vi "CircularBuffer.SetSize.vi"(8 "error in (no error)":errorcluster, 10 "BufferSize":i32=1, 11 "CircularBuffer":refnum<class "CircularBuffer.lvclass">) -> (0 "error out":errorcluster, 3 "CircularBuffer out":refnum<class "CircularBuffer.lvclass">)   [LabVIEW 2013, in "CircularBuffer.lvclass"]
doc: "---------------------------------------------------------------\nJKI State Machine Objects™\nhttp://jki.net/state-machine-objects/\nCopyright (C) 2005-2015, JKI <info@jki.net>\nALL RIGHTS RESERVEDJKI State Machine Objects (SMO) 1.0.0.5\nJKI - JKI\nCopyright (c) 2016, JKI"
uses:
  CircularBuffer.lvclass
  types/type/type.lvclass
panel:
  # "For instructions on how to use the JKI State Machine Objects, examples and video tutorials, visit:\nhttp://jki.net/state-machine-objects/\n\nJKI State Machine Objects™\nhttp://jki.net/state-machine-objects/\nCopyright (C) 2005-2015, JKI <info@jki.net>\nALL RIGHTS RESERVED"
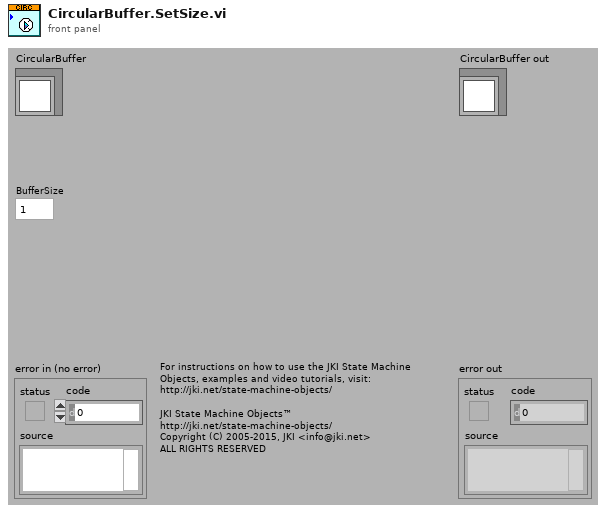
[diagram p1: front panel]
types:
  T1 = typedef "CircularBuffer.lvclass/PrivateData--Ref.ctl" = refnum<data-value>
  T2 = typedef "CircularBuffer.lvclass/PrivateData--Cluster.ctl" = cluster{"Public Events":T3, "Protected Events":T4, "Private Events":T5, "BufferSize":i32, "CurrentElement":i32, "Elements":refnum<data-value>[], "type":refnum<class "type.lvclass">}
  T3 = typedef "CircularBuffer.lvclass/PublicEvents--Cluster.ctl" = cluster{"Buffer Resize Event":refnum<user-event>}
  T4 = typedef "CircularBuffer.lvclass/ProtectedEvents--Cluster.ctl" = cluster{"placeholder":refnum<user-event>}
  T5 = typedef "CircularBuffer.lvclass/PrivateEvents--Cluster.ctl" = cluster{"New Value":refnum<user-event>, "GetElement":refnum<user-event>}
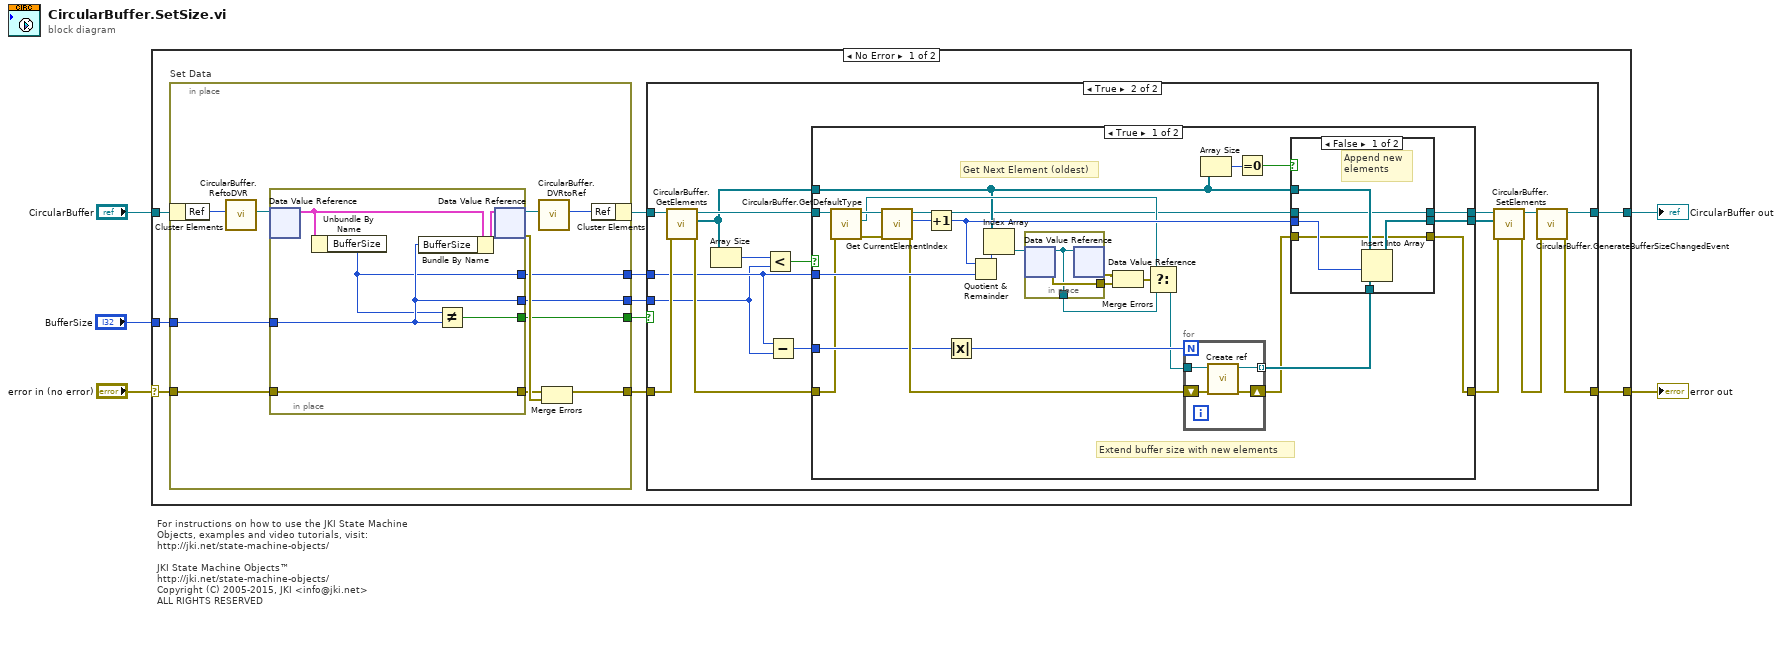
[diagram p0: block diagram]
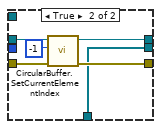
[diagram p3: hidden frame]
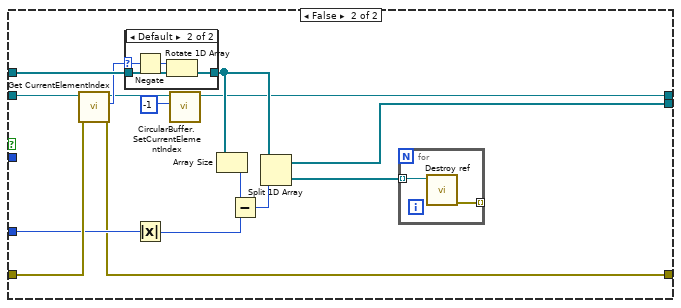
[diagram p4: hidden frame]
diagram:
  # "For instructions on how to use the JKI State Machine Objects, examples and video tutorials, visit:\nhttp://jki.net/state-machine-objects/\n\nJKI State Machine Objects™\nhttp://jki.net/state-machine-objects/\nCopyright (C) 2005-2015, JKI <info@jki.net>\nALL RIGHTS RESERVED"
  n1 = case shown="No Error" "error in (no error)" {
    selector: "error in (no error)" -> [w13 w120]
    tunnel: "CircularBuffer" -> [w14 w121]
    tunnel: [w11 w120] -> w4
    tunnel: [w9 w121] -> w3
    tunnel: "BufferSize" -> [w15 _]
    frame No Error {
      n2 = in-place "Set Data" {
        in-place-border: w13 -> [w113]
        in-place-border: [w110] -> w8
        in-place-border: w15 -> [w109]
        in-place-border: [w108] -> w12
        in-place-border: [w103] -> w7
        in-place-border: [w102] -> w6
        n3 = in-place-cluster #1(w14) -> ("Ref"=w107:u32)
        n4 = call "CircularBuffer.ReftoDVR.vi"("Ref"=w107) -> ("Ref"=w106:T1)  [unwired: 10 in]
        n5 = in-place {
          in-place-border: w113 -> [w119]
          in-place-border: [w119] -> w111
          in-place-border: w109 -> [w116]
          in-place-border: [w116] -> w108
          in-place-border: [w115] -> w103
          in-place-border: [w114] -> w102
          n6 = in-place-dvr #2(w106) -> (w117:T2)  [unwired: 1 out]
          n7 = Unbundle By Name(w117) -> ("BufferSize"=w114:i32)
          n8 = Bundle By Name(cluster=w117, "BufferSize"=w116) -> (w118:T2)
          n9 = Not Equal?(x=w114, y=w116) -> (x != y?=w115:bool)
          n10 = in-place-dvr #2(w118) -> (w105:T1, w112:errorcluster)
        }
        n11 = call "CircularBuffer.DVRtoRef.vi"("Ref"=w105) -> ("Ref"=w104:u32)  [unwired: 10 in]
        n12 = Merge Errors(w111, w112) -> (w110:errorcluster)
        n13 = in-place-cluster #1("Ref"=w104) -> (w10:refnum<class "CircularBuffer.lvclass">)
      }
      n14 = case shown="True" w7 {
        tunnel: w12 -> [_ w23]
        tunnel: [w16 w33] -> w11
        tunnel: w10 -> [w17 w32]
        tunnel: [w17 w34] -> w9
        tunnel: w8 -> [w16 w30]
        tunnel: w6 -> [_ w24]
        frame False {
        }
        frame True {
          n15 = call "CircularBuffer.GetElements.vi"("error in (no error)"=w30, "CircularBuffer in"=w32) -> ("error out"=w27:errorcluster, "Elements"=w25:refnum<data-value>[], "CircularBuffer out"=w31:refnum<class "CircularBuffer.lvclass">)  [unwired: 7 in]
          n16 = Array Size(array=w25) -> (size(s)=w29:i32)
          n17 = Less?(x=w29, y=w23) -> (x < y?=w28:bool)
          n18 = Subtract(x=w24, y=w23) -> (x-y=w22:i32)
          n19 = case shown="True" w28 {
            tunnel: [w39 w81] -> w26
            tunnel: w31 -> [w52 w94]
            tunnel: [w35 w83] -> w20
            tunnel: w27 -> [w50 w93]
            tunnel: w25 -> [w42 w91]
            tunnel: w24 -> [w61 _]
            tunnel: w22 -> [w57 w92]
            tunnel: [w55 w85] -> w21
            frame True {
              # "Get Next Element (oldest)"
              # "Extend buffer size with new elements"
              n20 = call "CircularBuffer.GetDefaultType.vi"("error in (no error)"=w50, "CircularBuffer"=w52) -> ("error out"=w49:errorcluster, "type"=w44:refnum<class "type.lvclass">, "CircularBuffer out"=w51:refnum<class "CircularBuffer.lvclass">)  [unwired: 7 in]
              n21 = call "Get CurrentElementIndex.vi"("error in (no error)"=w49, "CircularBuffer"=w51) -> ("error out"=w58:errorcluster, "Current Element index"=w53:i32, "CircularBuffer out"=w38:refnum<class "CircularBuffer.lvclass">)  [unwired: 7 in]
              n22 = Increment(x=w53) -> (x+1=w56:i32)
              n23 = Absolute Value(x=w57) -> (abs(x)=w54:i32)
              n24 = Quotient & Remainder(x=w56, y=w61) -> (x-y*floor(x/y)=w60:i32)  [unwired: 1 out]
              n25 = Index Array(array=w42, index=w60) -> (element=w59:refnum<data-value>)
              n26 = in-place {
                in-place-border: [w79] -> w47
                in-place-border: [w78] -> w45
                n27 = in-place-dvr #3(w59) -> (w78:refnum<class "type.lvclass">, w79:errorcluster)
                n28 = in-place-dvr #3(w78) -> (w48:errorcluster)  [unwired: 1 out]
              }
              n29 = Merge Errors(w48, w47) -> (w46:errorcluster)
              n30 = Select(t=w44, s=w46, f=w45) -> (s? t:f=w43:refnum<class "type.lvclass">)
              n31 = for {
                N: w54 -> [_]
                tunnel: [w75] -> w37 mode=indexing
                shift-right: [w76] -> w36
                shift-left: w58 -> [w77]
                tunnel: w43 -> [w74]
                n32 = call "Create ref.vi"("error in (no error)"=w77, "type in"=w74) -> ("error out"=w76:errorcluster, "data value reference"=w75:refnum<data-value>)  [unwired: 8 in]
              }
              n33 = Array Size(array=w42) -> (size(s)=w41:i32)
              n34 = Equal To 0?(x=w41) -> (x = 0?=w40:bool)
              n35 = case shown="False" w40 {
                tunnel: w56 -> [w67 _]
                tunnel: w37 -> [w66 w68]
                tunnel: [w65 w68] -> w55
                tunnel: w42 -> [w64 _]
                tunnel: [w63 w71] -> w39
                tunnel: w38 -> [w63 w72]
                tunnel: w36 -> [w62 w70]
                tunnel: [w62 w69] -> w35
                frame False {
                  # "Append new\nelements"
                  n36 = Insert Into Array(array=w64, index=w67, new element=w66) -> (w65:refnum<data-value>[])
                }
                frame True {
                  n37 = call "CircularBuffer.SetCurrentElementIndex.vi"("error in (no error)"=w70, "Index"=-1, "CircularBuffer"=w72) -> ("error out"=w69:errorcluster, "CircularBuffer out"=w71:refnum<class "CircularBuffer.lvclass">)  [unwired: 7 in]
                }
              }
            }
            frame False {
              n38 = call "Get CurrentElementIndex.vi"("error in (no error)"=w93, "CircularBuffer"=w94) -> ("error out"=w83:errorcluster, "Current Element index"=w90:i32, "CircularBuffer out"=w82:refnum<class "CircularBuffer.lvclass">)  [unwired: 7 in]
              n39 = case shown="Default" w90 {
                selector: w90 -> [_ w99]
                tunnel: w91 -> [w97 w101]
                tunnel: [w97 w98] -> w89
                frame -1 {
                }
                frame Default {
                  n40 = Negate(x=w99) -> (-x=w100:i32)
                  n41 = Rotate 1D Array(1:w101, 2:w100) -> (0:w98:refnum<data-value>[])
                }
              }
              n42 = Absolute Value(x=w92) -> (abs(x)=w87:i32)
              n43 = call "CircularBuffer.SetCurrentElementIndex.vi"("Index"=-1, "CircularBuffer"=w82) -> ("CircularBuffer out"=w81:refnum<class "CircularBuffer.lvclass">)  [unwired: 8 in, 1 out]
              n44 = Array Size(array=w89) -> (size(s)=w88:i32)
              n45 = Subtract(x=w88, y=w87) -> (x-y=w86:i32)
              n46 = Split 1D Array(array=w89, index=w86) -> (first subarray=w85:refnum<data-value>[], second subarray=w84:refnum<data-value>[])
              n47 = for {
                tunnel: w84 -> [w96] mode=indexing
                tunnel: [w95] -> _ mode=indexing
                n48 = call "Destroy ref.vi"("data value reference"=w96) -> ("error out"=w95:errorcluster)  [unwired: 10 in]
              }
            }
          }
          n49 = call "CircularBuffer.SetElements.vi"("error in (no error)"=w20, "Elements"=w21, "CircularBuffer in"=w26) -> ("error out"=w18:errorcluster, "CircularBuffer out"=w19:refnum<class "CircularBuffer.lvclass">)  [unwired: 7 in]
          n50 = call "CircularBuffer.GenerateBufferSizeChangedEvent.vi"("error in (no error)"=w18, "CircularBuffer in"=w19) -> ("error out"=w33:errorcluster, "CircularBuffer out"=w34:refnum<class "CircularBuffer.lvclass">)  [unwired: 8 in]
        }
      }
    }
    frame Error {
    }
  }
  "error out" <- w4
  "CircularBuffer out" <- w3
